vi "2photocell+ledcontrol+sum.vi"() -> ()   [LabVIEW 2016]
uses:
  <vilib>/LabVIEW Interface for Arduino/LabVIEW Interface for Arduino.lvlib
  <vilib>/ptbypt/NI_PtbyPt.lvlib
panel:
  in  "stop":bool
  in  "Tab Control":enum32{"Page 1", "Page 2"}(tab)
  out "LUX":dbl
  out "Voltage":dbl(knob) scale=0.0..5.0
  out "Filtered x":dbl format="%0.2f"
  in  "br_coef":dbl
  in  "thrs low":i32=1
  in  "thrs high":i32=4
  in  "Slide 3":dbl(slide) min=0.0 max=255.0 scale=0.0..255.0
  in  "Slide 2":dbl(slide) min=0.0 max=255.0 scale=0.0..255.0
  in  "Slide":dbl(slide) min=0.0 max=255.0 scale=0.0..255.0
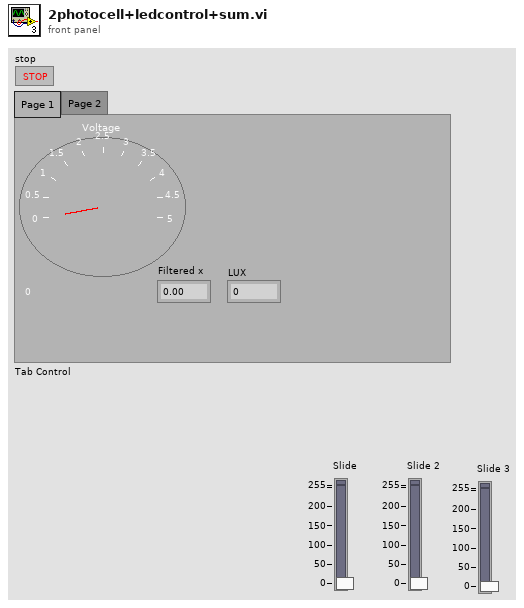
[diagram p1: front panel]
types:
  T1 = typedef "LabVIEW Interface for Arduino.lvlib/Arduino Resource.ctl" = cluster{"VISA resource":refnum<visa-resource-name>, "Board Type":T2, "Connection Type":enum8{"USB / Serial"}, "Bytes Per Packet (15)":u8}
  T2 = typedef "LabVIEW Interface for Arduino.lvlib/Board Type.ctl" = enum16{"Uno", "Dimuelanove w/Atmega 328", "Mega 2560"}
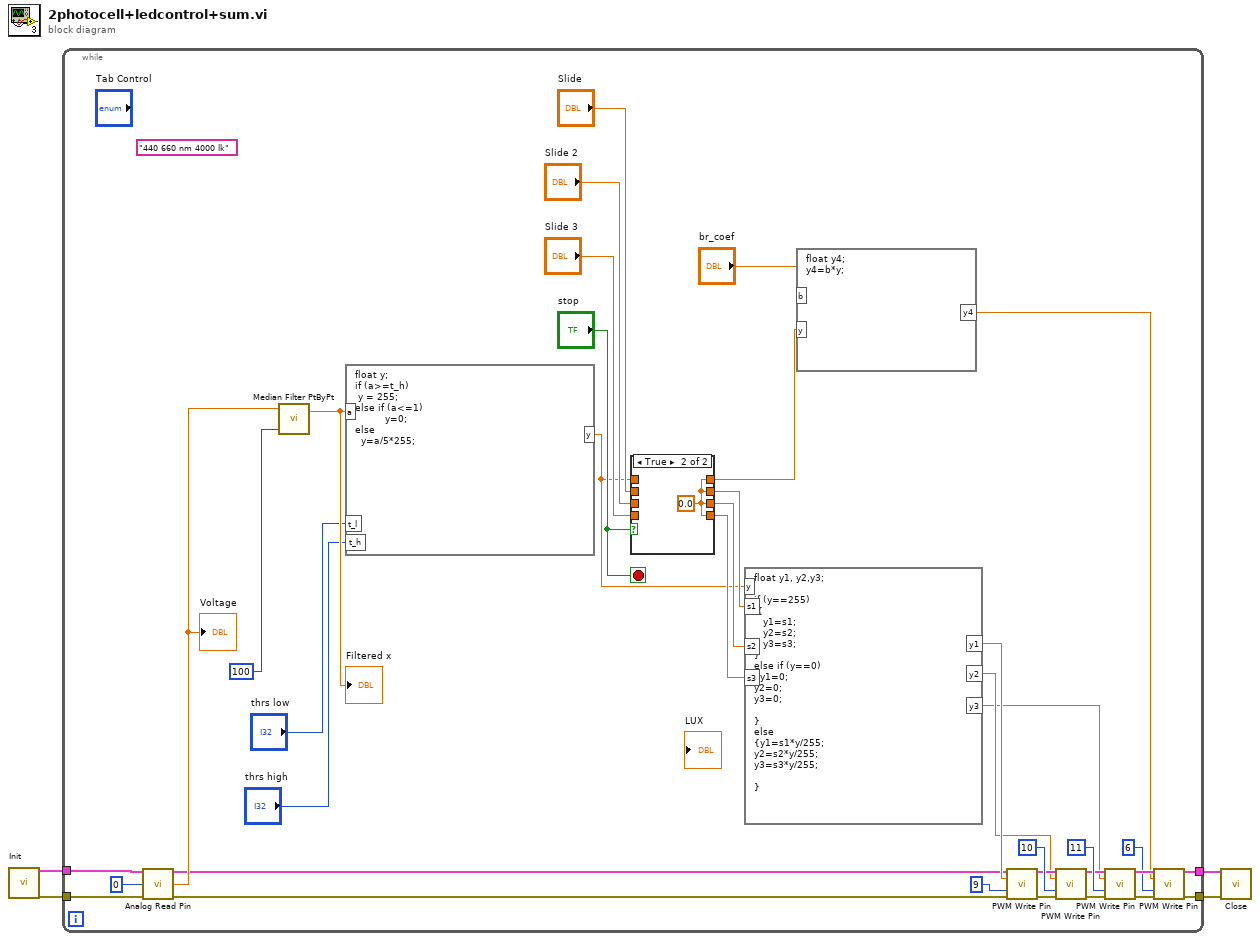
[diagram p0: block diagram]
diagram:
  n1 = call <vilib>:"Init.vi"() -> ("Arduino Resource"=w3:T1, "error out"=w4:errorcluster)  [unwired: 18 in]
  n2 = while {
    tunnel: w4 -> [w39]
    tunnel: w3 -> [w37]
    tunnel: [w14] -> w2
    tunnel: [w13] -> w1
    stop <- "stop" stop-if-true
    (unwired) "440 660 nm 4000 lk"
    n3 = call <vilib>:"Analog Read Pin.vi"("Arduino Resource"=w37, "Analog Input Pin (0)"=u8 0, "error in"=w39) -> ("Arduino Resource"=w6:T1, "Voltage"=w36:dbl, "error out"=w5:errorcluster)  [unwired: 10 in]
    "Voltage" <- w36
    n4 = call <vilib>:"Median Filter PtByPt.vi"("rank"=100, "x"=w36) -> ("Filtered x"=w34:dbl)  [unwired: 2 in, 1 out]
    "Filtered x" <- w34
    n5 = formula code="float y;\nif (a>=t_h)\n y = 255;\nelse if (a<=1)\n          y=0;\nelse\n  y=a/5*255;"("a"=w34, "t_l"="thrs low", "t_h"="thrs high") -> ("y"=w10:dbl)
    n6 = case shown="True" "stop" {
      tunnel: "Slide 2" -> [w44 _]
      tunnel: [w44 w45] -> w20
      tunnel: "Slide 3" -> [w43 _]
      tunnel: [w43 w45] -> w19
      tunnel: "Slide" -> [w42 _]
      tunnel: [w42 w45] -> w21
      tunnel: w10 -> [w41 _]
      tunnel: [w41 w45] -> w8
      frame False {
      }
      frame True {
        w45 = 0.0 ("Slide 2")
      }
    }
    n7 = formula code="float y1, y2,y3;\n\nif (y==255)\n {\n   y1=s1;\n   y2=s2;\n   y3=s3;\n}\nelse if (y==0)\n{y1=0;\ny2=0;\ny3=0;\n\n}\nelse \n{y1=s1*y/255;\ny2=s2*y/255;\ny3=s3*y/255;\n\n}"("s1"=w21, "s2"=w20, "s3"=w19, "y"=w10) -> ("y1"=w18:dbl, "y2"=w17:dbl, "y3"=w16:dbl)
    n8 = formula code="float y4;\ny4=b*y;"("b"="br_coef", "y"=w8) -> ("y4"=w7:dbl)
    n9 = call <vilib>:"PWM Write Pin.vi"("Arduino Resource"=w6, "Duty Cycle (0 - 255)"=w18, "PWM Pin (3)"=u8 9, "error in"=w5) -> ("Arduino Resource"=w27:T1, "error out"=w23:errorcluster)  [unwired: 10 in]
    n10 = call <vilib>:"PWM Write Pin.vi"("Arduino Resource"=w27, "Duty Cycle (0 - 255)"=w17, "PWM Pin (3)"=u8 10, "error in"=w23) -> ("Arduino Resource"=w26:T1, "error out"=w22:errorcluster)  [unwired: 10 in]
    n11 = call <vilib>:"PWM Write Pin.vi"("Arduino Resource"=w26, "Duty Cycle (0 - 255)"=w16, "PWM Pin (3)"=u8 11, "error in"=w22) -> ("Arduino Resource"=w15:T1, "error out"=w12:errorcluster)  [unwired: 10 in]
    n12 = call <vilib>:"PWM Write Pin.vi"("Arduino Resource"=w15, "Duty Cycle (0 - 255)"=w7, "PWM Pin (3)"=u8 6, "error in"=w12) -> ("Arduino Resource"=w14:T1, "error out"=w13:errorcluster)  [unwired: 10 in]
  }
  n13 = call <vilib>:"Close.vi"("Arduino Resource"=w2, "error in"=w1) -> ()  [unwired: 13 in, 1 out]
